vi "Write Ignore First Update.vi"(8 "error in (no error)":errorcluster, 10 "Ignore First Update":bool, 11 "CS++PVMonitor in":refnum<class "CS++PVMonitor.lvclass">) -> (0 "error out":errorcluster, 3 "CS++PVMonitor out":refnum<class "CS++PVMonitor.lvclass">)   [LabVIEW 2015, in "CS++PVMonitor.lvlib" / "CS++PVMonitor.lvclass"]
uses:
  CS++PVMonitor.lvclass
  CS++PVMonitor.lvclass/CS++PVMonitor.ctl
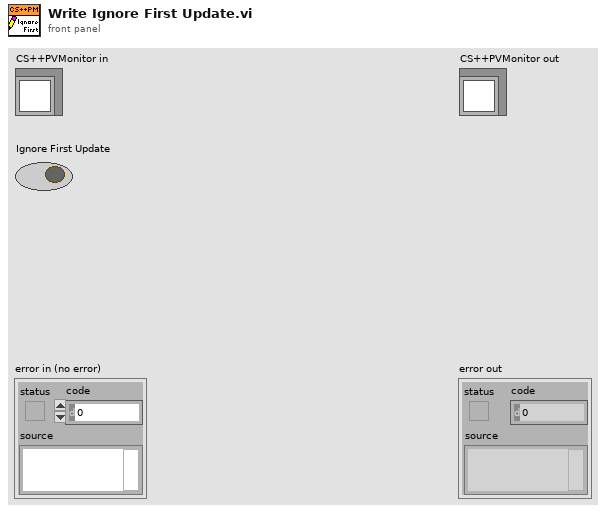
[diagram p1: front panel]
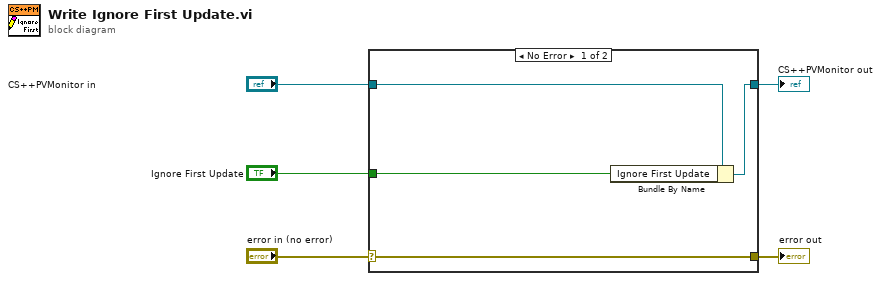
[diagram p0: block diagram]
diagram:
  n1 = case shown="No Error" "error in (no error)" {
    selector: "error in (no error)" -> [w9 w10]
    tunnel: [w9 w10] -> w4
    tunnel: [w7 w11] -> w2
    tunnel: "CS++PVMonitor in" -> [w8 w11]
    tunnel: "Ignore First Update" -> [w6 _]
    frame No Error {
      n2 = Bundle By Name(cluster=w8, "Ignore First Update"=w6) -> (w7:refnum<class "CS++PVMonitor.lvclass">)
    }
    frame Error {
    }
  }
  "error out" <- w4
  "CS++PVMonitor out" <- w2
